vi "Set APU.vi"(8 "error in (no error)":errorcluster, 10 "APU Settings":T1, 11 "APU Node":refnum<k24>) -> (0 "error out":errorcluster, 3 "APU Node":refnum<k24>)   [LabVIEW 2015, in "Engine Simulation Toolkit SysDef API.lvlib"]
uses:
  Engine Simulation Toolkit SysDef API.lvlib
  NationalInstruments.VeriStand.SystemDefinitionAPI
  APU Settings.ctl
  Shared/Properties.vi
  Shared/Constants and GUIDs.vi
  <vilib>/NI Veristand/Custom Device API/Set Item Property (Double).vi
  <vilib>/NI Veristand/Custom Device Tools/Custom Device Utility Library/NI VeriStand - Search for Item by Name.vi
  <vilib>/NI Veristand/Custom Device API/Set Item Property (Boolean).vi
  Shared/Engine Simulation Toolkit Shared.lvlib
  <vilib>/NI VeriStand/Custom Device API/Custom Device API.lvlib
  <vilib>/NI VeriStand/Custom Device Tools/Custom Device Utility Library/Custom Device Utility Library.lvlib
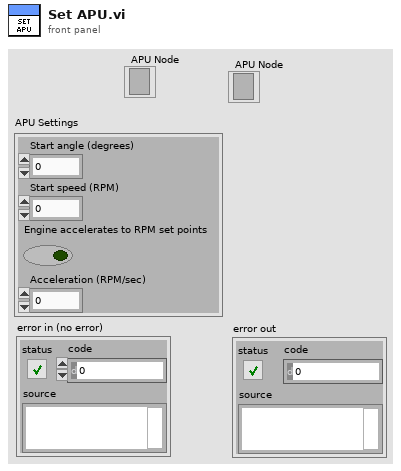
[diagram p1: front panel]
types:
  T1 = typedef "Engine Simulation Toolkit SysDef API.lvlib/APU Settings.ctl" = cluster{"Start angle (degrees)":dbl, "Start speed (RPM)":dbl, "Engine accelerates to RPM set points":bool, "Acceleration (RPM/sec)":dbl}
  T2 = typedef "Engine Simulation Toolkit Shared.lvlib/Channel.ctl" = cluster{"Name":string, "Units":string, "Default":dbl, "Description":string, "Scalable":bool}
  T3 = typedef "Custom Device API.lvlib/Custom Device Item Ref.ctl" = u64
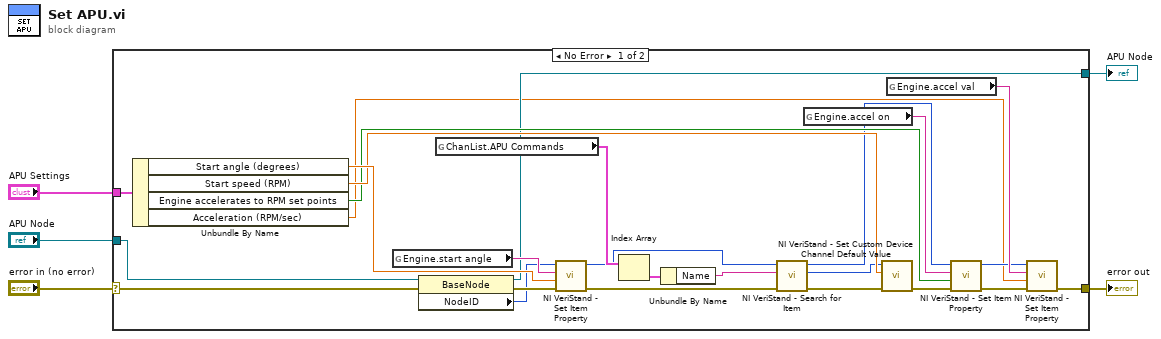
[diagram p0: block diagram]
diagram:
  n1 = case shown="No Error" "error in (no error)" {
    selector: "error in (no error)" -> [w16 w32]
    tunnel: [w25 w32] -> w5
    tunnel: "APU Node" -> [w17 w31]
    tunnel: [w14 w31] -> w2
    tunnel: "APU Settings" -> [w21 _]
    frame No Error {
      n2 = Unbundle By Name(w21) -> ("Start angle (degrees)"=w20:dbl, "Start speed (RPM)"=w19:dbl, "Engine accelerates to RPM set points"=w18:bool, "Acceleration (RPM/sec)"=w6:dbl)
      n3 = global read "Properties.vi" "Engine.start angle"() -> (w29:string)
      n4 = property class="BaseNode"(reference=w17, error in=w16) -> (reference out=w14:refnum<k24>, error out=w15:errorcluster, "NodeID"=w13:u64)
      n5 = global read "Constants and GUIDs.vi" "ChanList.APU Commands"() -> (w23:T2[])
      n6 = call-poly <vilib>:"NI VeriStand - Set Item Property.vi"("error in (no error)"=w15, "Value"=w20, "Property Name"=w29, "Item Ref in"=w13) -> ("error out"=w10:errorcluster, "Item Ref out"=w12:T3)  [unwired: 5 in, 1 out]
      n7 = Index Array(array=w23) -> (element=w24:T2)  [unwired: 1 in]
      n8 = Unbundle By Name(w24) -> ("Name"=w11:string)
      n9 = call-poly <vilib>:"NI VeriStand - Search for Item.vi"("error in"=w10, "Item Name"=w11, "Section Ref in"=w12) -> ("error out"=w9:errorcluster, "Item Ref"=w8:T3, "Section Ref out"=w7:T3)  [unwired: 5 in, 1 out]
      n10 = global read "Properties.vi" "Engine.accel on"() -> (w30:string)
      n11 = call <vilib>:"NI VeriStand - Set Custom Device Channel Default Value.vi"("error in (no error)"=w9, "Default Value"=w19, "Channel Ref in"=w8) -> ("error out"=w27:errorcluster)  [unwired: 7 in, 1 out]
      n12 = global read "Properties.vi" "Engine.accel val"() -> (w28:string)
      n13 = call-poly <vilib>:"NI VeriStand - Set Item Property.vi"("error in (no error)"=w27, "Value"=w18, "Property Name"=w30, "Item Ref in"=w7) -> ("error out"=w26:errorcluster, "Item Ref out"=w22:T3)  [unwired: 5 in, 1 out]
      n14 = call-poly <vilib>:"NI VeriStand - Set Item Property.vi"("error in (no error)"=w26, "Value"=w6, "Property Name"=w28, "Item Ref in"=w22) -> ("error out"=w25:errorcluster)  [unwired: 5 in, 2 out]
    }
    frame Error {
    }
  }
  "error out" <- w5
  "APU Node" <- w2
